vi "schedulerActionSelector.vi"(9 "Read Default Schedule":bool, 10 "Update Scheduler":bool, 11 "Clear Scheduler":bool) -> (2 "Scheduler Action":dbl)   [LabVIEW 2018]
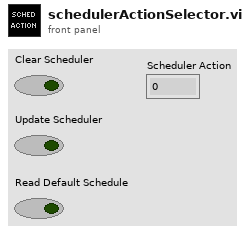
[diagram p1: front panel]
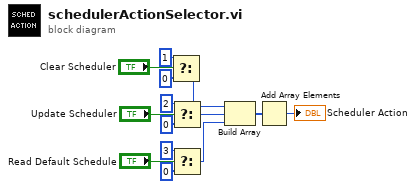
[diagram p0: block diagram]
diagram:
  n1 = Select(t=1, s="Clear Scheduler", f=0) -> (s? t:f=w4:i32)
  n2 = Select(t=2, s="Update Scheduler", f=0) -> (s? t:f=w5:i32)
  n3 = Select(t=3, s="Read Default Schedule", f=0) -> (s? t:f=w3:i32)
  n4 = Build Array(w4, w5, w3) -> (w2:i32[])
  n5 = Add Array Elements(numeric array=w2) -> (sum=→"Scheduler Action":i32)
